vi "Send Event.vi"(8 "Error in":errorcluster, 9 "Data":variant, 10 "Cmd":string, 11 "Event Ref":refnum<user-event>) -> (0 "Error out":errorcluster, 3 "Event Ref out":refnum<user-event>)   [LabVIEW 2018, in "Event Messaging.lvlib"]
uses:
  Event Messaging.lvlib
  Type Defs/Event Message--cluster.ctl
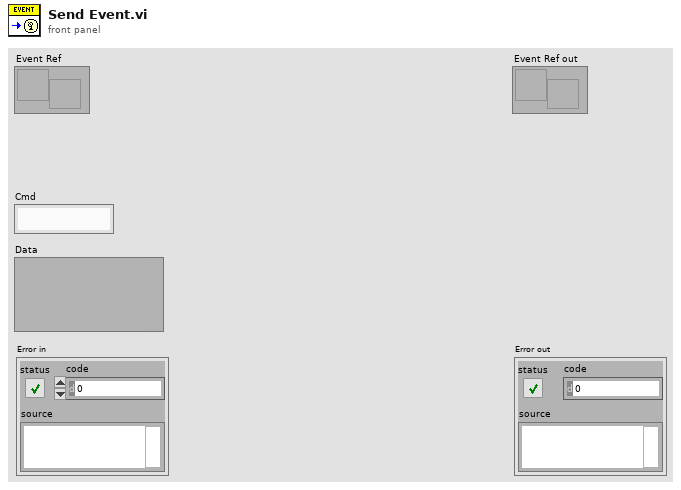
[diagram p1: front panel]
types:
  T1 = typedef "Event Messaging.lvlib/Event Message--cluster.ctl" = cluster{"Cmd":string, "Data":variant}
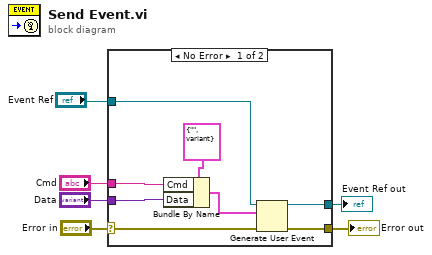
[diagram p0: block diagram]
diagram:
  n1 = case shown="No Error" "Error in" {
    selector: "Error in" -> [w12 w16]
    tunnel: [w11 w16] -> w5
    tunnel: "Data" -> [w10 _]
    tunnel: "Cmd" -> [w9 _]
    tunnel: "Event Ref" -> [w8 w15]
    tunnel: [w7 w15] -> w1
    frame No Error {
      n2 = Bundle By Name(cluster=T1 {"Cmd"="", "Data"=variant} ("Message"), "Cmd"=w9, "Data"=w10) -> (w14:T1)
      n3 = Generate User Event(user event=w8, event data cluster=w14, error in=w12) -> (user event out=w7:refnum<user-event>, error out=w11:errorcluster)  [unwired: 1 in]
    }
    frame Error {
    }
  }
  "Error out" <- w5
  "Event Ref out" <- w1
